vi "Generator Driver Template 1.vi"() -> ()   [LabVIEW 2019]
uses:
  subVIs/Revidyne Generator.lvlib
panel:
  in  "stop":bool
  out "Waveform Chart":dbl(graph)
  in  "VISA resource name":refnum<visa-resource-name>
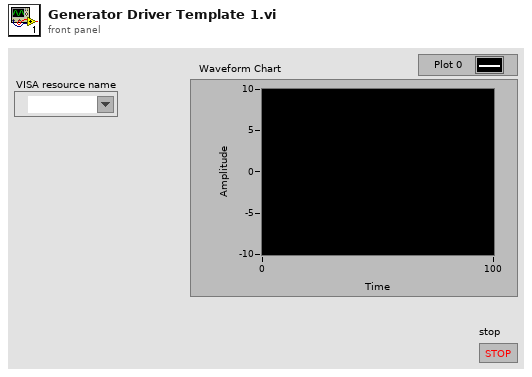
[diagram p1: front panel]
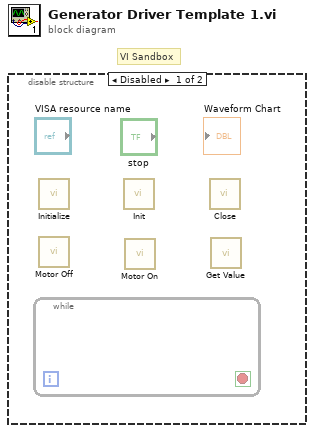
[diagram p0: block diagram]
diagram:
  # "VI Sandbox"
  n1 = disable-structure shown="Disabled" {
    frame Disabled {
      n2 = while {
        stop <- _ stop-if-true
      }
      n3 = call "Initialize.vi"() -> ()  [unwired: 10 in, 2 out]
      n4 = call "Motor Off.vi"() -> ()  [unwired: 10 in, 2 out]
      n5 = call "Init.vi"() -> ()  [unwired: 10 in, 2 out]
      n6 = call "Motor On.vi"() -> ()  [unwired: 10 in, 2 out]
      n7 = call "Close.vi"() -> ()  [unwired: 11 in, 1 out]
      n8 = call "Get Value.vi"() -> ()  [unwired: 9 in, 3 out]
    }
    frame Enabled {
    }
  }
